vi "Signal-exit.vi"(8 "error in (no error)":errorcluster, 11 "ModComm in":T1) -> (0 "error out":errorcluster, 3 "ModComm out":T1)   [LabVIEW 2013, in "Server.lvlib" / "Server.lvclass"]
uses:
  Server.lvclass
  Object-reference.ctl
  Server.lvclass/Server.ctl
  Read Exit.vi
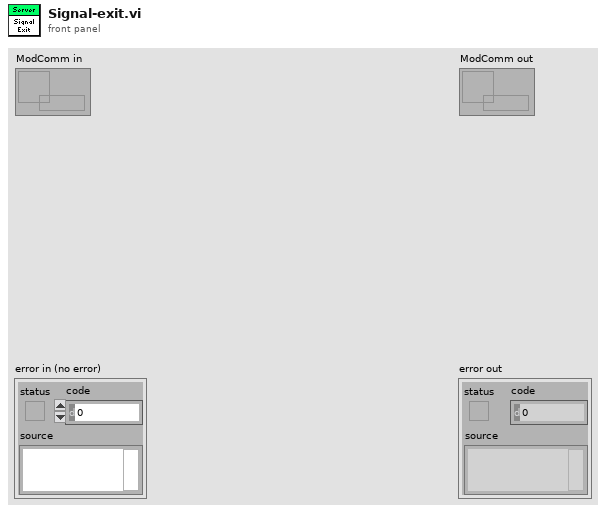
[diagram p1: front panel]
types:
  T1 = typedef "Server.lvlib/Server.lvclass/Object-reference.ctl" = refnum<data-value>
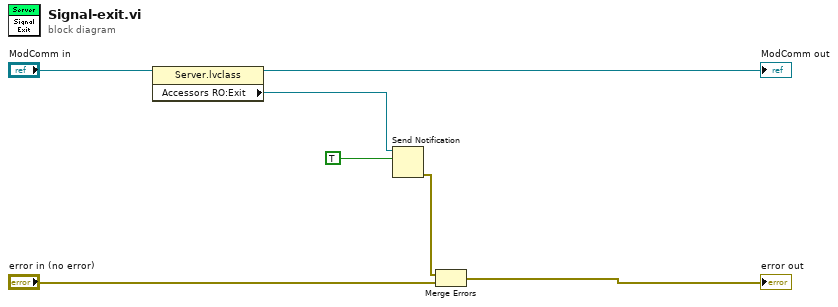
[diagram p0: block diagram]
diagram:
  n1 = property class="Server.lvclass"(reference="ModComm in") -> (reference out=→"ModComm out":T1, "Accessors RO:Exit"=w5:refnum<notifier>)  [unwired: 1 in, 1 out]
  n2 = Send Notification(notification=TRUE, notifier=w5) -> (error out=w1:errorcluster)  [unwired: 1 in, 1 out]
  n3 = Merge Errors(w1, "error in (no error)") -> (→"error out":errorcluster)
